vi "d1000 get command pos.vi"(11 "axis":i16) -> (3 "function return":i32)   [LabVIEW 2019, in "Dmc1000.lvlib"]
doc: "DMC1000_API long WINAPI d1000_get_command_pos(short axis);"
uses:
  Dmc1000.lvlib
  Dmc1000.dll
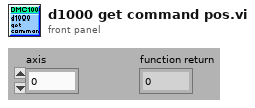
[diagram p1: front panel]
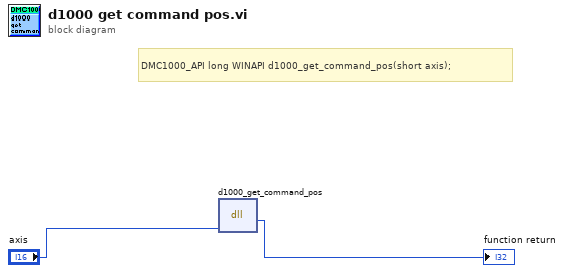
[diagram p0: block diagram]
diagram:
  # "DMC1000_API long WINAPI d1000_get_command_pos(short axis);"
  n1 = dll-call lib="C:/Users/VIC/Desktop/Standar Program/System/LLB/DMC1000B/Dmc1000.*" fn="d1000_get_command_pos"("axis"="axis") -> (→"function return":i32)  [unwired: 4 in, 2 out]
